vi "FTW-JSON-Native-GetFlattenedValue.vi"(0 "JSON Element":string, 5 "Element Data Name":string, 7 "LabVIEW Type":T1, 9 "Element Default Value":variant, 11 "error in":errorcluster) -> (4 "Flattened Value":string, 15 "error out":errorcluster)   [LabVIEW 2013]
uses:
  Reflection/FTW-Reflection-Types.ctl
panel:
  # "Inputs"
  # "Outputs"
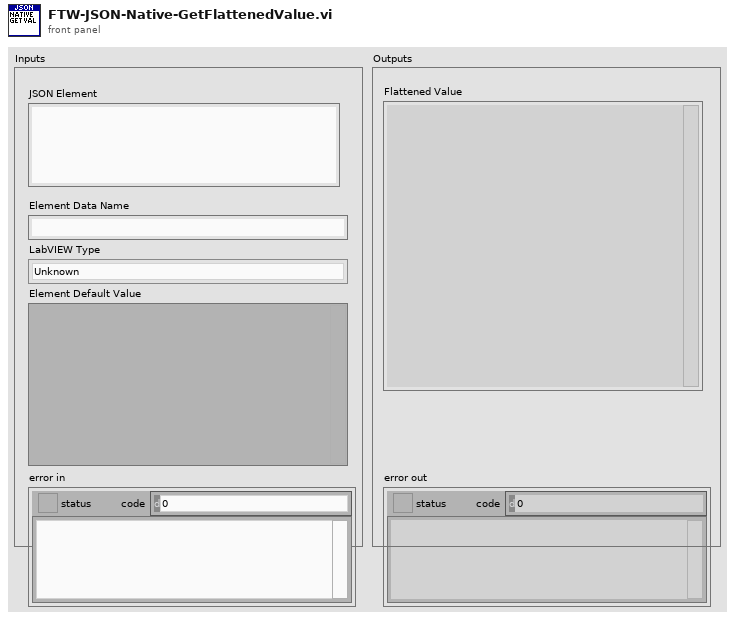
[diagram p1: front panel]
types:
  T1 = typedef "FTW-Reflection-Types.ctl" = enum16{"Unknown", "Void", "Array", "Cluster", "LVObject", "Boolean", "I8", "I16", "I32", "I64", "U8", "U16", "U32", "U64", "SGL", "DBL", "EXT", "CSG", "CDB", "CXT", "FXP", "EnumU8", "EnumU16", "EnumU32", "EnumU64", "SGLwithUnit", "DBLwithUnit", "EXTwithUnit", "CSGwithUnit", "CDBwithUnit", "CXTwithUnit", "String", "Path", "Picture", "Tag", "LVVariant", "Timestamp", "WaveformI8", "WaveformI16", "WaveformI32", "WaveformI64", "WaveformU8", "WaveformU16", "WaveformU32", "WaveformU64", "WaveformSGL", "WaveformDBL", "WaveformEXT", "WaveformCSG", "WaveformCDB", "WaveformCXT", "WaveformDigital", "WaveformUnknownType", "DigitalData", "DynamicData", "ExternalData", "FileByteStream", "TDMStream", "dotNET", "ActiveX", "VIServerReference", "VIReference", "ApplicationInstance", "Menu", "ConnectionDataSocket", "ConnectionVISA", "ConnectionBluetooth", "ConnectionIrDA", "ConnectionTCP", "ConnectionUDP", "ConnectionHTTPClient", "ConnectionFTP", "Occurrence", "Notifier", "Queue", "Rendezvous", "Semaphore", "RTFIFO", "EventPublisher", "EventRegistration", "EventCallback", "DataValueReference", "GenericClass", "GenericClassTag", "GenericClassDeepCopy", "GenericClassFlattened", "GenericClassTagFlattened", "GenericReferenceType", "WindowsRegistry", "OverloadedDatalogRef", "ReferenceUnknownType"}
  T2 = cluster{"Element Name":string, "Element Type":T1, "Element Value":variant}[]
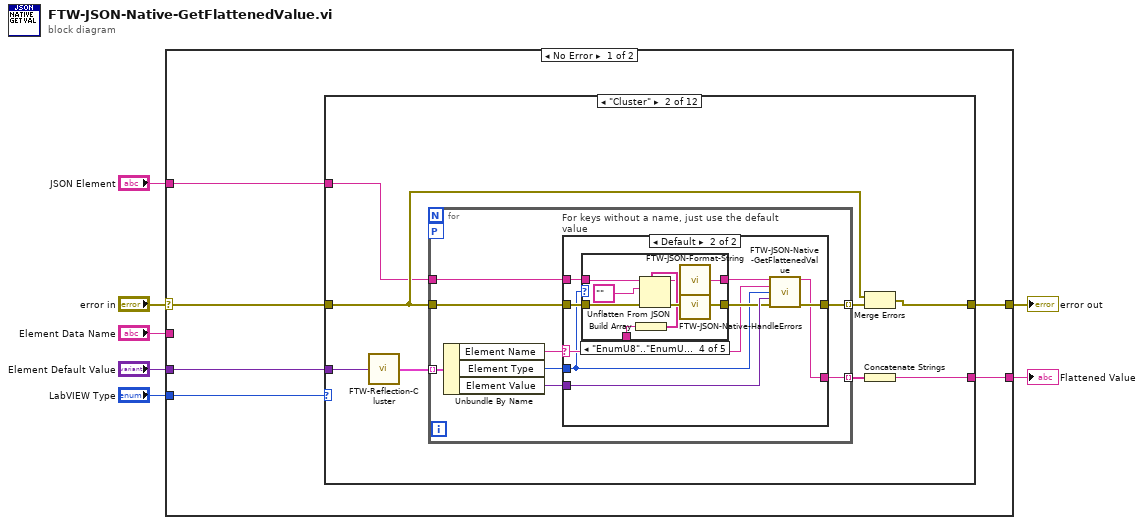
[diagram p0: block diagram]
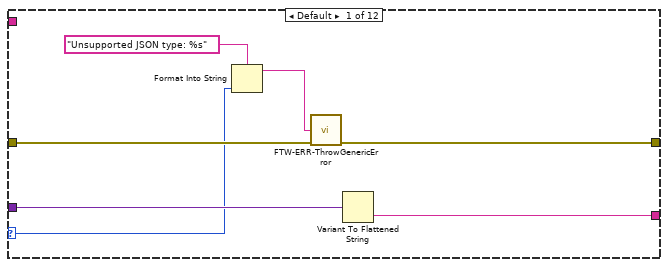
[diagram p2: hidden frame]
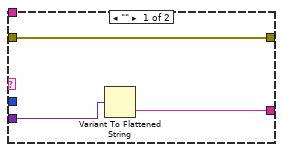
[diagram p3: hidden frame]
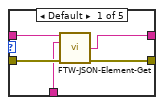
[diagram p4: hidden frame]
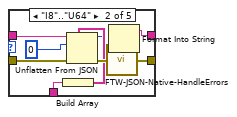
[diagram p5: hidden frame]
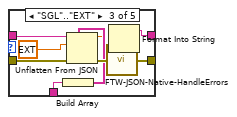
[diagram p6: hidden frame]
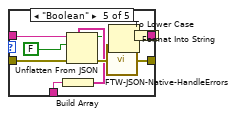
[diagram p7: hidden frame]
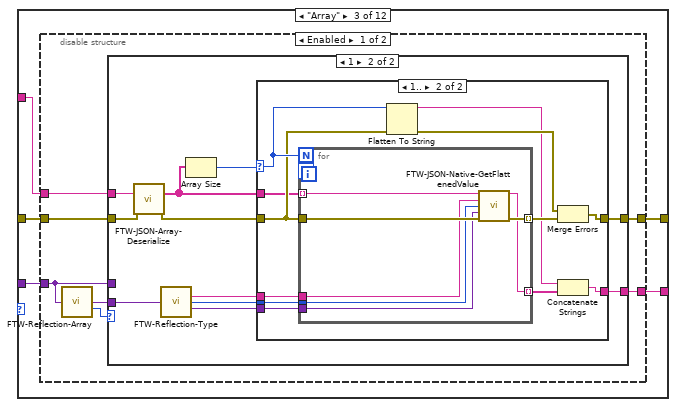
[diagram p8: hidden frame]
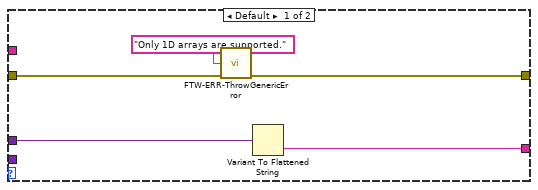
[diagram p9: hidden frame]
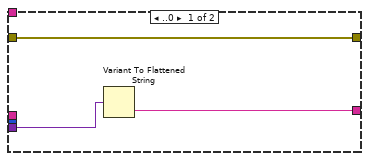
[diagram p10: hidden frame]
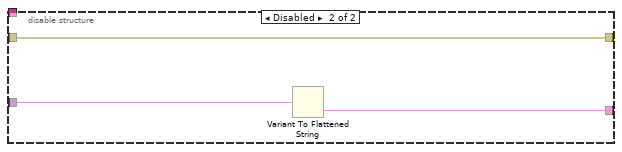
[diagram p11: hidden frame]
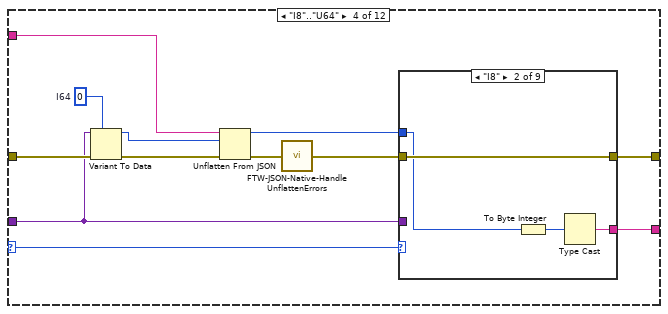
[diagram p12: hidden frame]
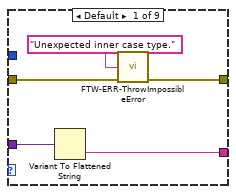
[diagram p13: hidden frame]
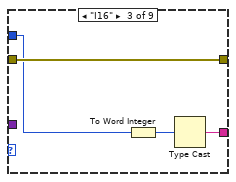
[diagram p14: hidden frame]
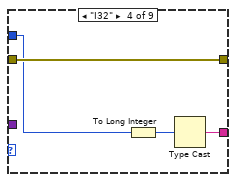
[diagram p15: hidden frame]
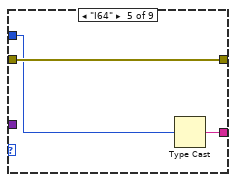
[diagram p16: hidden frame]
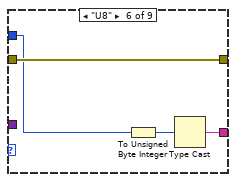
[diagram p17: hidden frame]
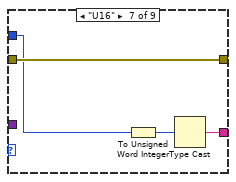
[diagram p18: hidden frame]
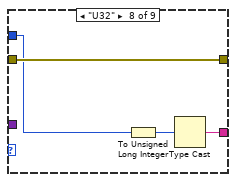
[diagram p19: hidden frame]
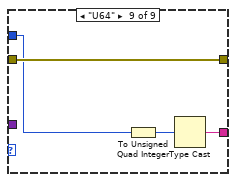
[diagram p20: hidden frame]
diagram:
  n1 = case shown="No Error" "error in" {
    selector: "error in" -> [w9 w349]
    tunnel: [w13 w349] -> w7
    tunnel: "JSON Element" -> [w8 _]
    tunnel: [w12 w347] -> w5
    tunnel: "LabVIEW Type" -> [w11 _]
    tunnel: "Element Default Value" -> [w10 w348]
    tunnel: "Element Data Name" -> [_ _]
    frame No Error {
      n2 = case shown="\"Cluster\"" w11 {
        selector: w11 -> [w14 _ _ w153 w200 w245 _ _ _ _ _ _]
        tunnel: [w17 w26 w93 w152 w199 w244 w263 w283 w296 w304 w326 w337] -> w13
        tunnel: [w15 w27 w94 w154 w201 w246 w273 w284 w297 w308 w327 w345] -> w12
        tunnel: w9 -> [w18 w25 w92 w155 w198 w240 w268 w278 w291 w299 w317 w346]
        tunnel: w10 -> [w16 w28 w95 w150 w195 w239 w267 w279 w292 w300 w316 w339]
        tunnel: w8 -> [_ w24 w91 w145 w193 w236 w264 w275 w288 w305 w319 w338]
        frame Default {
          n3 = Format Into String(format string="Unsupported JSON type: %s", w14) -> (resulting string=w20:string)  [unwired: 2 in, 1 out]
          n4 = call "FTW-ERR-ThrowGenericError.vi"("Error Message"=w20, "error in"=w18) -> ("error out"=w17:errorcluster)  [unwired: 13 in]
          n5 = Variant To Flattened String(Variant=w16) -> (data string=w15:string)  [unwired: 1 out]
        }
        frame "Cluster" {
          n6 = call "FTW-Reflection-Cluster.vi"("Cluster"=w28) -> ("Cluster Elements"=w23:T2)  [unwired: 14 in]
          n7 = for {
            tunnel: w23 -> [w35] mode=indexing
            tunnel: [w32] -> w22 mode=indexing
            tunnel: w25 -> [w36]
            tunnel: [w30] -> w21 mode=indexing
            workers-P: _ -> [_]
            tunnel: w24 -> [w29]
            n8 = Unbundle By Name(w35) -> ("Element Name"=w34:string, "Element Type"=w31:T1, "Element Value"=w33:variant)
            n9 = case "For keys without a name, just use the default value" shown="Default" w34 {
              selector: w34 -> [_ w42]
              tunnel: w36 -> [w37 w45]
              tunnel: w33 -> [w39 w46]
              tunnel: [w38 w47] -> w32
              tunnel: w31 -> [_ w40]
              tunnel: [w37 w48] -> w30
              tunnel: w29 -> [_ w43]
              frame "" {
                n10 = Variant To Flattened String(Variant=w39) -> (data string=w38:string)  [unwired: 1 out]
              }
              frame Default {
                n11 = case shown="\"EnumU8\"..\"EnumU64\", \"String\"" w40 {
                  tunnel: w45 -> [w53 w62 w71 w80 w90]
                  tunnel: [w52 w54 w63 w72 w81] -> w44
                  tunnel: w43 -> [w51 w60 w69 w78 w88]
                  tunnel: w42 -> [w50 w58 w67 w76 w86]
                  tunnel: [w49 w55 w64 w73 w82] -> w41
                  frame Default {
                    n12 = call "FTW-JSON-Element-Get.vi"("JSON Opject"=w51, "Key"=w50, "error in"=w53) -> ("Element"=w49:string, "error out"=w52:errorcluster)  [unwired: 10 in, 1 out]
                  }
                  frame "I8".."U64" {
                    n13 = Build Array(w58) -> (w57:string[])
                    n14 = Unflatten From JSON(path=w57, JSON string=w60, type and defaults=i64 0, error in (no error)=w62) -> (value=w56:i64, error out=w61:errorcluster)  [unwired: 3 in]
                    n15 = call "FTW-JSON-Native-HandleErrors.vi"("error in"=w61) -> ("error out"=w54:errorcluster)  [unwired: 14 in]
                    n16 = Format Into String(w56) -> (resulting string=w55:string)  [unwired: 3 in, 1 out]
                  }
                  frame "SGL".."EXT" {
                    n17 = Build Array(w67) -> (w66:string[])
                    n18 = Unflatten From JSON(path=w66, JSON string=w69, type and defaults=ext 0.0, error in (no error)=w71) -> (value=w65:ext, error out=w70:errorcluster)  [unwired: 3 in]
                    n19 = call "FTW-JSON-Native-HandleErrors.vi"("error in"=w70) -> ("error out"=w63:errorcluster)  [unwired: 14 in]
                    n20 = Format Into String(w65) -> (resulting string=w64:string)  [unwired: 3 in, 1 out]
                  }
                  frame "EnumU8".."EnumU64", "String" {
                    n21 = Build Array(w76) -> (w75:string[])
                    n22 = Unflatten From JSON(path=w75, JSON string=w78, type and defaults="", error in (no error)=w80) -> (value=w74:string, error out=w79:errorcluster)  [unwired: 3 in]
                    n23 = call "FTW-JSON-Format-String.vi"("LabVIEW String"=w74) -> ("JSON String"=w73:string)
                    n24 = call "FTW-JSON-Native-HandleErrors.vi"("error in"=w79) -> ("error out"=w72:errorcluster)  [unwired: 14 in]
                  }
                  frame "Boolean" {
                    n25 = Build Array(w86) -> (w85:string[])
                    n26 = Unflatten From JSON(path=w85, JSON string=w88, type and defaults=FALSE, error in (no error)=w90) -> (value=w84:bool, error out=w89:errorcluster)  [unwired: 3 in]
                    n27 = call "FTW-JSON-Native-HandleErrors.vi"("error in"=w89) -> ("error out"=w81:errorcluster)  [unwired: 14 in]
                    n28 = Format Into String(w84) -> (resulting string=w83:string)  [unwired: 3 in, 1 out]
                    n29 = To Lower Case(string=w83) -> (all lower case string=w82:string)
                  }
                }
                n30 = call "FTW-JSON-Native-GetFlattenedValue.vi"("JSON Element"=w41, "Element Data Name"=w42, "LabVIEW Type"=w40, "Element Default Value"=w46, "error in"=w44) -> ("Flattened Value"=w47:string, "error out"=w48:errorcluster)  [unwired: 9 in]
              }
            }
          }
          n31 = Merge Errors(w25, w21) -> (w26:errorcluster)
          n32 = Concatenate Strings(w22) -> (w27:string)
        }
        frame "Array" {
          n33 = disable-structure shown="Enabled" {
            disable-tunnel: w95 -> [w102 w142]
            disable-tunnel: [w101 w141] -> w94
            disable-tunnel: [w100 w143] -> w93
            disable-tunnel: w92 -> [w99 w143]
            disable-tunnel: w91 -> [w96 _]
            frame Enabled {
              n34 = call "FTW-Reflection-Array.vi"("Array"=w102) -> ("Default Array Element"=w98:variant, "Number of Dimensions"=w97:i32)  [unwired: 13 in]
              n35 = case shown="1" w97 {
                tunnel: [w104 w118] -> w101
                tunnel: [w105 w117] -> w100
                tunnel: w99 -> [w106 w111]
                tunnel: w98 -> [_ w116]
                tunnel: w102 -> [w103 _]
                tunnel: w96 -> [_ w112]
                frame Default {
                  n36 = call "FTW-ERR-ThrowGenericError.vi"("Error Message"="Only 1D arrays are supported.", "error in"=w106) -> ("error out"=w105:errorcluster)  [unwired: 13 in]
                  n37 = Variant To Flattened String(Variant=w103) -> (data string=w104:string)  [unwired: 1 out]
                }
                frame 1 {
                  n38 = call "FTW-JSON-Array-Deserialize.vi"("Array of JSON Objects"=w112, "error in"=w111) -> ("JSON Elements"=w109:string[], "error out"=w110:errorcluster)  [unwired: 11 in, 1 out]
                  n39 = call "FTW-Reflection-Type.vi"("Anything"=w116) -> ("Data Name"=w113:string, "LabVIEW Type"=w115:T1, "Variant Type and Value"=w114:variant)  [unwired: 12 in]
                  n40 = Array Size(array=w109) -> (size(s)=w108:i32)
                  n41 = case shown="1.." w108 {
                    selector: w108 -> [_ w127]
                    tunnel: [w121 w133] -> w118
                    tunnel: [w119 w132] -> w117
                    tunnel: w110 -> [w119 w124]
                    tunnel: w115 -> [_ w130]
                    tunnel: w114 -> [w120 w129]
                    tunnel: w113 -> [_ w123]
                    tunnel: w109 -> [_ w122]
                    frame ..0 {
                      n42 = Variant To Flattened String(Variant=w120) -> (data string=w121:string)  [unwired: 1 out]
                    }
                    frame 1.. {
                      n43 = for {
                        N: w127 -> [_]
                        workers-P: _ -> [_]
                        tunnel: w124 -> [w140]
                        tunnel: [w139] -> w131 mode=indexing
                        tunnel: w130 -> [w136]
                        tunnel: w129 -> [w137]
                        tunnel: [w138] -> w128 mode=indexing
                        tunnel: w123 -> [w135]
                        tunnel: w122 -> [w134] mode=indexing
                        n44 = call "FTW-JSON-Native-GetFlattenedValue.vi"("JSON Element"=w134, "Element Data Name"=w135, "LabVIEW Type"=w136, "Element Default Value"=w137, "error in"=w140) -> ("Flattened Value"=w138:string, "error out"=w139:errorcluster)  [unwired: 9 in]
                      }
                      n45 = Flatten To String(anything=w127, error in (no error)=w124) -> (data string=w125:string, error out=w126:errorcluster)  [unwired: 2 in, 1 out]
                      n46 = Merge Errors(w126, w131) -> (w132:errorcluster)
                      n47 = Concatenate Strings(w125, w128) -> (w133:string)
                    }
                  }
                }
              }
            }
            frame Disabled {
              n48 = Variant To Flattened String(Variant=w142) -> (data string=w141:string)  [unwired: 1 out]
            }
          }
        }
        frame "I8".."U64" {
          w149 = i64 0  # I64
          n49 = Variant To Data(error in=w155, type=w149, Variant=w150) -> (data=w148:i64, error out=w151:errorcluster)
          n50 = Unflatten From JSON(JSON string=w145, type and defaults=w148, error in (no error)=w151) -> (value=w147:i64, error out=w146:errorcluster)  [unwired: 4 in]
          n51 = call "FTW-JSON-Native-HandleUnflattenErrors.vi"("error in"=w146) -> ("error out"=w144:errorcluster)  [unwired: 14 in]
          n52 = case shown="\"I8\"" w153 {
            tunnel: [w159 w164 w168 w172 w175 w179 w183 w187 w191] -> w152
            tunnel: w144 -> [w160 w164 w168 w172 w175 w179 w183 w187 w191]
            tunnel: w147 -> [_ w162 w166 w170 w173 w177 w181 w185 w189]
            tunnel: [w156 w163 w167 w171 w174 w178 w182 w186 w190] -> w154
            tunnel: w150 -> [w157 _ _ _ _ _ _ _ _]
            frame Default {
              n53 = Variant To Flattened String(Variant=w157) -> (data string=w156:string)  [unwired: 1 out]
              n54 = call "FTW-ERR-ThrowImpossibleError.vi"("Reason this error should never happen"="Unexpected inner case type.", "error in"=w160) -> ("error out"=w159:errorcluster)  [unwired: 13 in]
            }
            frame "I8" {
              n55 = To Byte Integer(number=w162) -> (8bit integer=w161:i8)
              n56 = Type Cast(x=w161) -> (*(type *) &x=w163:string)  [unwired: 1 in]
            }
            frame "I16" {
              n57 = To Word Integer(number=w166) -> (16bit integer=w165:i16)
              n58 = Type Cast(x=w165) -> (*(type *) &x=w167:string)  [unwired: 1 in]
            }
            frame "I32" {
              n59 = To Long Integer(number=w170) -> (32bit integer=w169:i32)
              n60 = Type Cast(x=w169) -> (*(type *) &x=w171:string)  [unwired: 1 in]
            }
            frame "I64" {
              n61 = Type Cast(x=w173) -> (*(type *) &x=w174:string)  [unwired: 1 in]
            }
            frame "U8" {
              n62 = To Unsigned Byte Integer(number=w177) -> (unsigned 8bit integer=w176:u8)
              n63 = Type Cast(x=w176) -> (*(type *) &x=w178:string)  [unwired: 1 in]
            }
            frame "U16" {
              n64 = To Unsigned Word Integer(number=w181) -> (unsigned 16bit integer=w180:u16)
              n65 = Type Cast(x=w180) -> (*(type *) &x=w182:string)  [unwired: 1 in]
            }
            frame "U32" {
              n66 = To Unsigned Long Integer(number=w185) -> (unsigned 32bit integer=w184:u32)
              n67 = Type Cast(x=w184) -> (*(type *) &x=w186:string)  [unwired: 1 in]
            }
            frame "U64" {
              n68 = To Unsigned Quad Integer(1:w189) -> (0:w188:u64)
              n69 = Type Cast(x=w188) -> (*(type *) &x=w190:string)  [unwired: 1 in]
            }
          }
        }
        frame "EnumU8".."EnumU64" {
          n70 = call "FTW-Reflection-Enum.vi"("Enum"=w195) -> ("Selected Item"=w196:string)  [unwired: 12 in, 2 out]
          n71 = Unflatten From JSON(JSON string=w193, type and defaults=w196, error in (no error)=w198) -> (value=w197:string, error out=w194:errorcluster)  [unwired: 4 in]
          n72 = call "FTW-JSON-Native-HandleUnflattenErrors.vi"("error in"=w194) -> ("error out"=w192:errorcluster)  [unwired: 14 in]
          n73 = case shown="\"EnumU8\"" w200 {
            tunnel: [w205 w213 w220 w227 w234] -> w199
            tunnel: w192 -> [w206 w213 w220 w227 w234]
            tunnel: w197 -> [_ w210 w217 w224 w233]
            tunnel: [w202 w209 w216 w223 w232] -> w201
            tunnel: w195 -> [w203 w212 w219 w226 w229]
            frame Default {
              n74 = Variant To Flattened String(Variant=w203) -> (data string=w202:string)  [unwired: 1 out]
              n75 = call "FTW-ERR-ThrowImpossibleError.vi"("Reason this error should never happen"="Unexpected inner case type.", "error in"=w206) -> ("error out"=w205:errorcluster)  [unwired: 13 in]
            }
            frame "EnumU8" {
              n76 = call "FTW-Reflection-Enum.vi"("Enum"=w212) -> ("Enum Items"=w211:string[])  [unwired: 12 in, 2 out]
              n77 = Search 1D Array(1D array=w211, element=w210) -> (index of element=w208:i32)  [unwired: 1 in]
              n78 = To Unsigned Byte Integer(number=w208) -> (unsigned 8bit integer=w207:u8)
              n79 = Type Cast(x=w207) -> (*(type *) &x=w209:string)  [unwired: 1 in]
            }
            frame "EnumU16" {
              n80 = call "FTW-Reflection-Enum.vi"("Enum"=w219) -> ("Enum Items"=w218:string[])  [unwired: 12 in, 2 out]
              n81 = Search 1D Array(1D array=w218, element=w217) -> (index of element=w215:i32)  [unwired: 1 in]
              n82 = To Unsigned Word Integer(number=w215) -> (unsigned 16bit integer=w214:u16)
              n83 = Type Cast(x=w214) -> (*(type *) &x=w216:string)  [unwired: 1 in]
            }
            frame "EnumU32" {
              n84 = call "FTW-Reflection-Enum.vi"("Enum"=w226) -> ("Enum Items"=w225:string[])  [unwired: 12 in, 2 out]
              n85 = Search 1D Array(1D array=w225, element=w224) -> (index of element=w222:i32)  [unwired: 1 in]
              n86 = To Unsigned Long Integer(number=w222) -> (unsigned 32bit integer=w221:u32)
              n87 = Type Cast(x=w221) -> (*(type *) &x=w223:string)  [unwired: 1 in]
            }
            frame "EnumU64" {
              n88 = call "FTW-Reflection-Enum.vi"("Enum"=w229) -> ("Enum Items"=w228:string[])  [unwired: 12 in, 2 out]
              n89 = Search 1D Array(1D array=w228, element=w233) -> (index of element=w231:i32)  [unwired: 1 in]
              n90 = To Unsigned Quad Integer(1:w231) -> (0:w230:u64)
              n91 = Type Cast(x=w230) -> (*(type *) &x=w232:string)  [unwired: 1 in]
            }
          }
        }
        frame "SGL".."EXT" {
          w242 = 0.0  # dbl
          n92 = Variant To Data(error in=w240, type=w242, Variant=w239) -> (data=w241:dbl, error out=w243:errorcluster)
          n93 = Unflatten From JSON(JSON string=w236, type and defaults=w241, error in (no error)=w243) -> (value=w238:dbl, error out=w237:errorcluster)  [unwired: 4 in]
          n94 = call "FTW-JSON-Native-HandleUnflattenErrors.vi"("error in"=w237) -> ("error out"=w235:errorcluster)  [unwired: 14 in]
          n95 = case shown="\"SGL\"" w245 {
            tunnel: [w250 w255 w258 w262] -> w244
            tunnel: w235 -> [w251 w255 w258 w262]
            tunnel: w238 -> [_ w252 w256 w260]
            tunnel: [w247 w254 w257 w261] -> w246
            tunnel: w239 -> [w248 _ _ _]
            frame Default {
              n96 = Variant To Flattened String(Variant=w248) -> (data string=w247:string)  [unwired: 1 out]
              n97 = call "FTW-ERR-ThrowImpossibleError.vi"("Reason this error should never happen"="Unexpected inner case type.", "error in"=w251) -> ("error out"=w250:errorcluster)  [unwired: 13 in]
            }
            frame "SGL" {
              n98 = To Single Precision Float(number=w252) -> (single precision float=w253:sgl)
              n99 = Type Cast(x=w253) -> (*(type *) &x=w254:string)  [unwired: 1 in]
            }
            frame "DBL" {
              n100 = Type Cast(x=w256) -> (*(type *) &x=w257:string)  [unwired: 1 in]
            }
            frame "EXT" {
              n101 = To Extended Precision Float(1:w260) -> (0:w259:ext)
              n102 = Type Cast(x=w259) -> (*(type *) &x=w261:string)  [unwired: 1 in]
            }
          }
        }
        frame "Timestamp" {
          w270 = 0.0  # dbl
          n103 = Variant To Data(error in=w268, type=w270, Variant=w267) -> (data=w269:dbl, error out=w271:errorcluster)
          n104 = Unflatten From JSON(JSON string=w264, type and defaults=w269, error in (no error)=w271) -> (value=w265:dbl, error out=w266:errorcluster)  [unwired: 4 in]
          n105 = call "FTW-JSON-Native-HandleUnflattenErrors.vi"("error in"=w266) -> ("error out"=w263:errorcluster)  [unwired: 14 in]
          n106 = To Time Stamp(1:w265) -> (0:w272:timestamp)
          n107 = Type Cast(x=w272) -> (*(type *) &x=w273:string)  [unwired: 1 in]
        }
        frame "String", "ConnectionVISA" {
          # "ignore path not found error\nand use default value"
          n108 = Variant To Data(error in=w278, type="", Variant=w279) -> (data=w280:string, error out=w282:errorcluster)
          n109 = Unflatten From JSON(JSON string=w275, type and defaults=w280, error in (no error)=w282) -> (value=w277:string, error out=w276:errorcluster)  [unwired: 4 in]
          n110 = call "FTW-JSON-Native-HandleUnflattenErrors.vi"("error in"=w276) -> ("error out"=w274:errorcluster)  [unwired: 14 in]
          n111 = Flatten To String(anything=w277, error in (no error)=w274) -> (data string=w284:string, error out=w283:errorcluster)  [unwired: 2 in, 1 out]
        }
        frame "Path" {
          # "ignore path not found error\nand use default value"
          n112 = Variant To Data(error in=w291, type=path "", Variant=w292) -> (data=w293:path, error out=w295:errorcluster)
          n113 = Path To String(path=w293) -> (string=w285:string)
          n114 = Unflatten From JSON(JSON string=w288, type and defaults=w285, error in (no error)=w295) -> (value=w290:string, error out=w289:errorcluster)  [unwired: 4 in]
          n115 = call "FTW-JSON-Native-HandleUnflattenErrors.vi"("error in"=w289) -> ("error out"=w287:errorcluster)  [unwired: 14 in]
          n116 = String To Path(string=w290) -> (path=w286:path)
          n117 = Flatten To String(anything=w286, error in (no error)=w287) -> (data string=w297:string, error out=w296:errorcluster)  [unwired: 2 in, 1 out]
        }
        frame "Picture" {
          # "ignore path not found error\nand use default value"
          n118 = Variant To Flattened String(Variant=w300) -> (data string=w298:string)  [unwired: 1 out]
          n119 = call "FTW-STR-Encode-Base64.vi"("Input"=w298, "Direction"=enum16{"Encode", "Decode"}."Encode") -> ("Output"=w301:string)
          n120 = Unflatten From JSON(JSON string=w305, type and defaults=w301, error in (no error)=w299) -> (value=w307:string, error out=w306:errorcluster)  [unwired: 4 in]
          n121 = call "FTW-JSON-Native-HandleUnflattenErrors.vi"("error in"=w306) -> ("error out"=w304:errorcluster)  [unwired: 14 in]
          n122 = call "FTW-STR-Encode-Base64.vi"("Input"=w307, "Direction"=enum16{"Encode", "Decode"}."Decode") -> ("Output"=w308:string)
        }
        frame "FileByteStream".."ConnectionDataSocket", "ConnectionBluetooth".."ReferenceUnknownType" {
          w325 = "0x%16x"  # Reference Format
          n123 = Variant To Flattened String(Variant=w316) -> (data string=w315:string)  [unwired: 1 out]
          n124 = Type Cast(type=refnum<k0> refnum, x=w315) -> (*(type *) &x=w313:refnum<k0>)
          n125 = Type Cast(type=i64 0 ("default value 1"), x=w313) -> (*(type *) &x=w311:i64)
          n126 = Format Into String(format string="0x%016x", w311) -> (resulting string=w309:string)  [unwired: 2 in, 1 out]
          n127 = Unflatten From JSON(JSON string=w319, type and defaults=w309, error in (no error)=w317) -> (value=w320:string, error out=w321:errorcluster)  [unwired: 4 in]
          n128 = call "FTW-JSON-Native-HandleUnflattenErrors.vi"("error in"=w321) -> ("error out"=w318:errorcluster)  [unwired: 14 in]
          n129 = Scan From String(format string=w325, input string=w320, error in=w318, default 1=i64 0 ("default value 1")) -> (error out=w323:errorcluster, output 1=w324:i64)  [unwired: 1 in, 2 out]
          n130 = case shown="No Error" w323 {
            selector: w323 -> [w328 _]
            tunnel: [w332 w335] -> w327
            tunnel: w324 -> [w331 _]
            tunnel: w316 -> [_ w336]
            tunnel: [w328 w334] -> w326
            frame No Error {
              n131 = Type Cast(type=refnum<k0> refnum, x=w331) -> (*(type *) &x=w330:refnum<k0>)
              n132 = Type Cast(x=w330) -> (*(type *) &x=w332:string)  [unwired: 1 in]
            }
            frame Error {
              n133 = Variant To Flattened String(Variant=w336) -> (data string=w335:string)  [unwired: 1 out]
              n134 = call "FTW-ERR-ThrowGenericError.vi"("Error Message"="Unexpected reference format.") -> ("error out"=w334:errorcluster)  [unwired: 14 in]
            }
          }
        }
        frame "Boolean" {
          n135 = Variant To Data(error in=w346, type=FALSE, Variant=w339) -> (data=w343:bool, error out=w340:errorcluster)
          n136 = Unflatten From JSON(JSON string=w338, type and defaults=w343, error in (no error)=w340) -> (value=w341:bool, error out=w342:errorcluster)  [unwired: 4 in]
          n137 = Type Cast(x=w341) -> (*(type *) &x=w345:string)  [unwired: 1 in]
          n138 = call "FTW-JSON-Native-HandleUnflattenErrors.vi"("error in"=w342) -> ("error out"=w337:errorcluster)  [unwired: 14 in]
        }
      }
    }
    frame Error {
      n139 = Variant To Flattened String(Variant=w348) -> (data string=w347:string)  [unwired: 1 out]
    }
  }
  "error out" <- w7
  "Flattened Value" <- w5
